vi "merFISH_save_embryo_position.vi"(6 "XY REF cluster":T1, 7 "queue ASI stage":refnum<queue>, 8 "error in":errorcluster, 9 "Image Dst":T2, 10 "Image contrast":cluster{i32, i32}, 11 "New Image":T2) -> (0 "error out":errorcluster, 3 "REF positions OUT":dbl[][](array[numeric]), 5 "XY positions OUT":dbl[][](array[numeric]))   [LabVIEW 2015]
uses:
  <vilib>/vision/Image Controls.llb/IMAQ Image.ctl
  CONTROLS/Q_ASI_stage_element.ctl
  GLOBAL/Global_ASI_stage.vi
panel:
  in  "Define REF":bool caption="Save X/Y position"
  in  "Define embryo":bool caption="Save X/Y position"
  in  "Embryo Pos 2":bool caption="Save X/Y position"
  in  "Embryo Pos 1":bool caption="Save X/Y position"
  out "XY positions":cluster{dbl[], dbl[]}[](graph)
  in  "stop":bool
  out "Intensity range":cluster{sgl, sgl}(slide) scale=0.0..16000.0
  out "Image":T2(plugin-control)
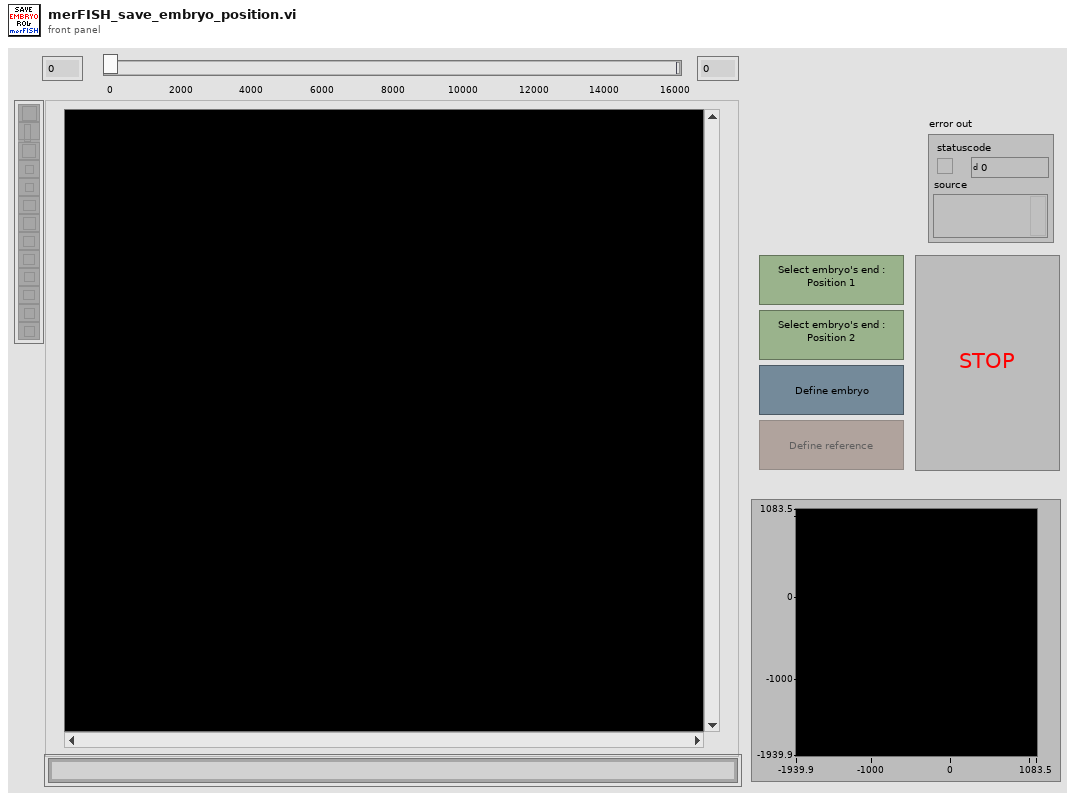
[diagram p1: front panel]
types:
  T1 = cluster{"XY positions":dbl[][], "REF positions":dbl[][]}
  T2 = typedef "IMAQ Image.ctl" = refnum<image>
  T3 = enum8{"Enabled", "Disabled", "Disabled and Grayed Out"}
  T4 = cluster{"Left":i32, "Top":i32, "Right":i32, "Bottom":i32}
  T5 = typedef "Q_ASI_stage_element.ctl" = cluster{"variant":variant, "Instruction":enum16{"ASI_idle", "ASI_initialize", "ASI_error", "ASI_security_stop", "ASI_read_XYZ", "ASI_up", "ASI_down", "ASI_left", "ASI_right", "ASI_save_XY", "ASI_move_to_XY", "ASI_brightfield", "ASI_init_scan", "ASI_init_merFISH", "ASI_move_to_XY_merFISH", "ASI_move_to_Z_merFISH", "ASI_init_autofocus_search_merFISH", "ASI_close_autofocus_search_merFISH", "ASI_adjust_piezo_autofocus_merFISH", "ASI_set_piezo_autofocus_to_reference_position_merFISH_TL", "ASI_close_merFISH", "ASI_stop"}}
  T6 = cluster{"Mean Value":sgl, "Standard Variation":sgl, "Minimal Value":sgl, "Maximal Value":sgl, "Area (calibrated)":sgl, "Area (pixels)":u32, "%":sgl, "Calibration Valid":bool}
  T7 = cluster{"Maximal Value":sgl, "Minimal Value":sgl}
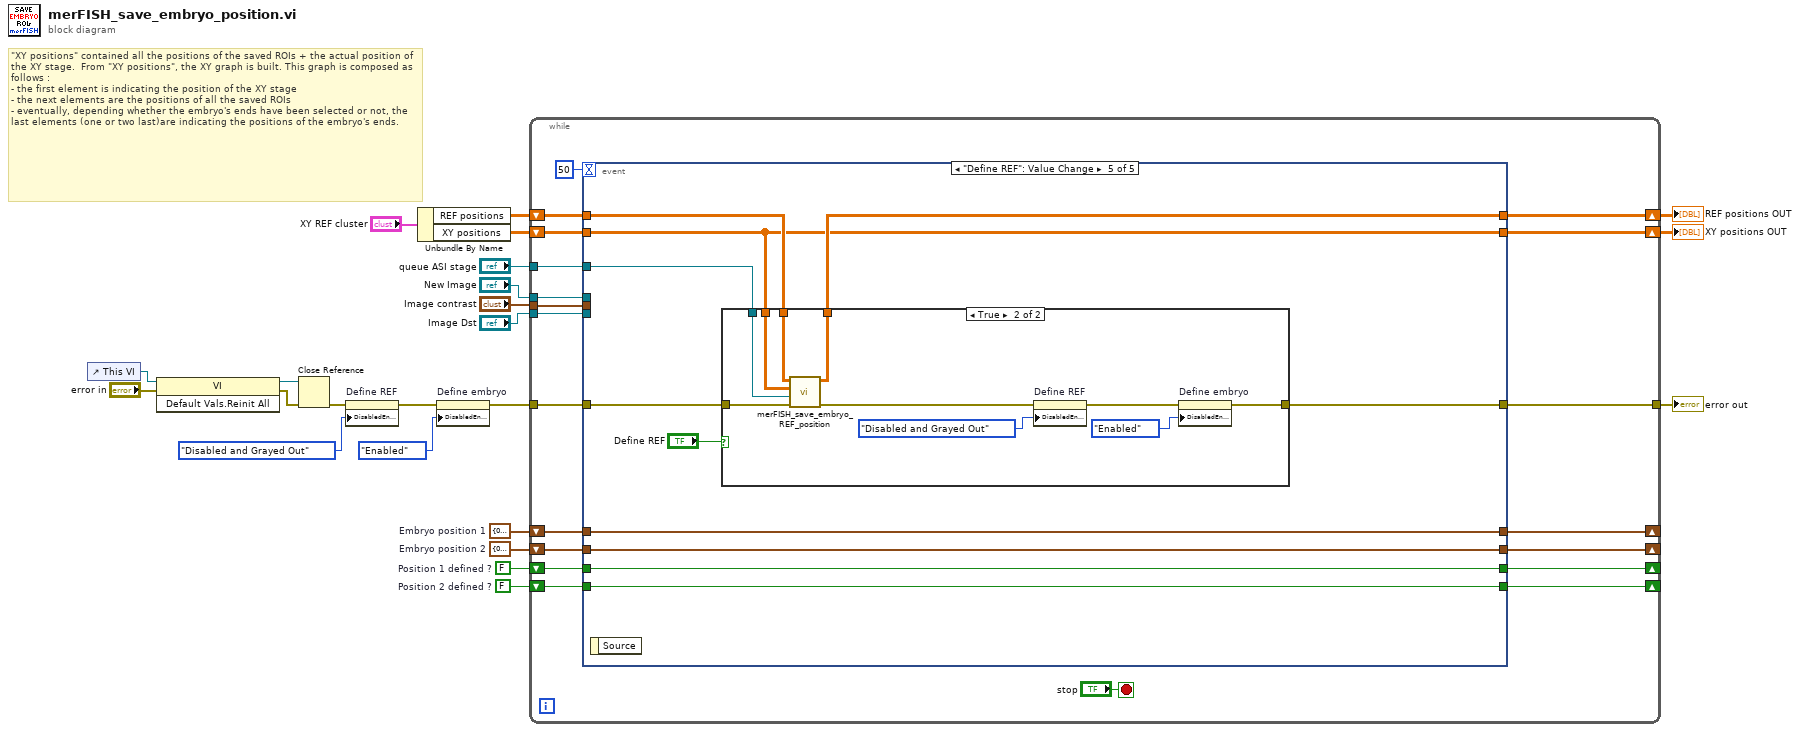
[diagram p0: block diagram]
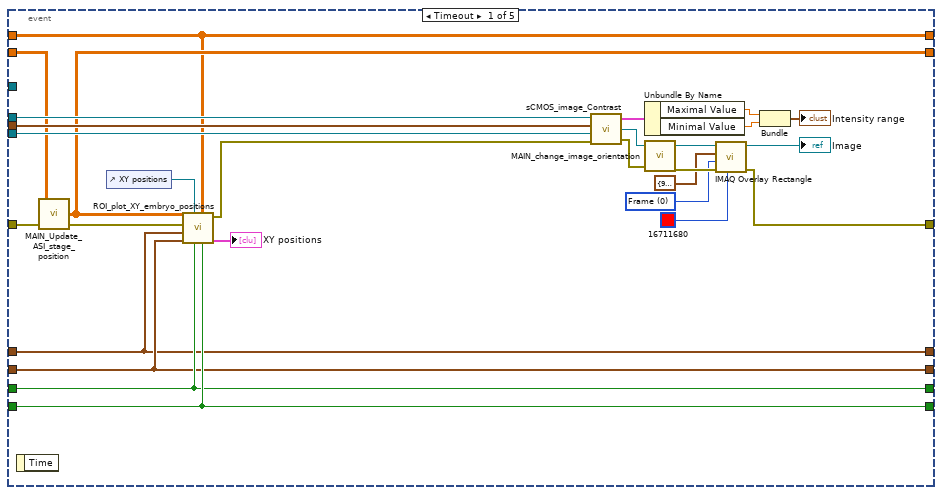
[diagram p2: hidden frame]
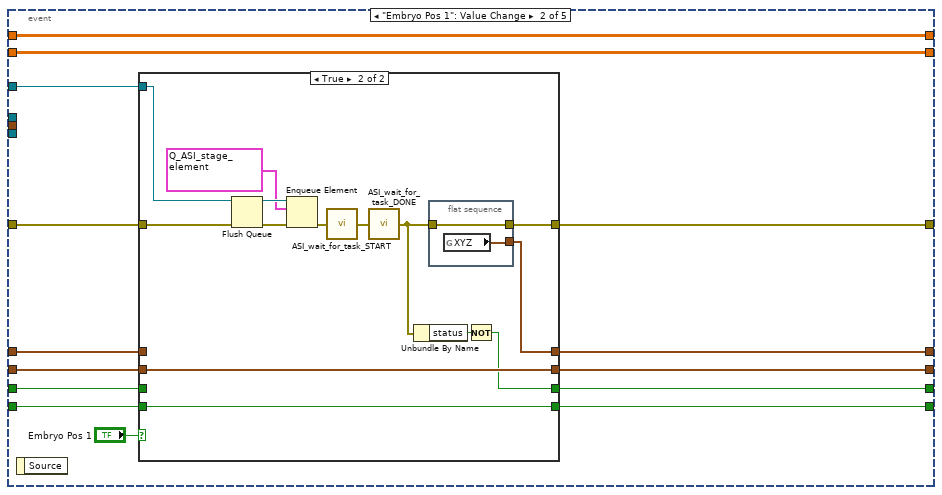
[diagram p3: hidden frame]
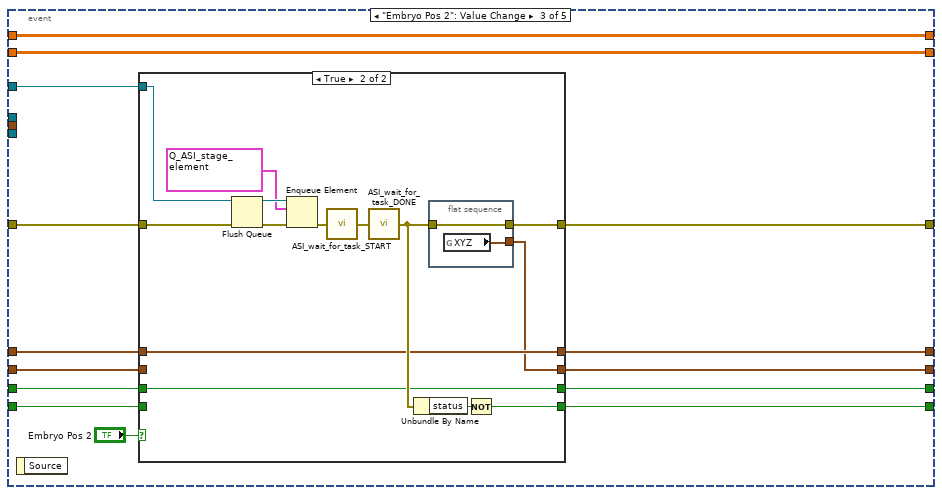
[diagram p5: hidden frame]
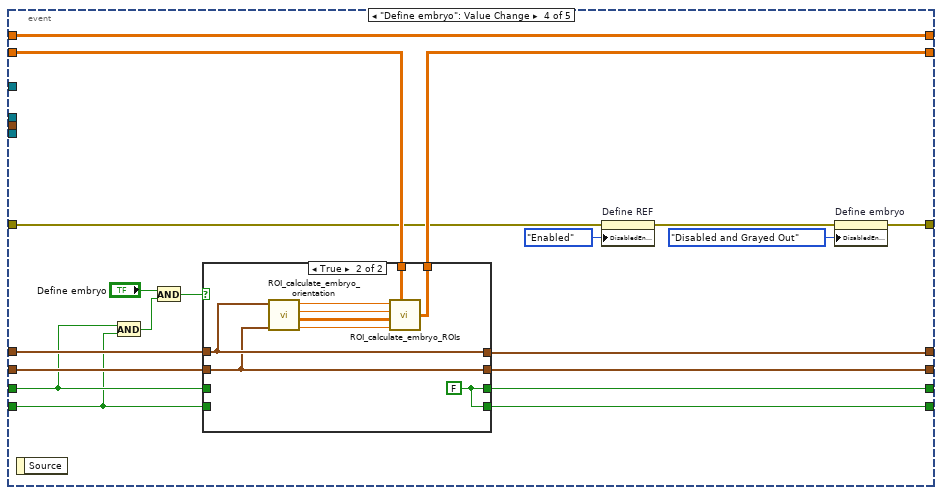
[diagram p7: hidden frame]
diagram:
  w12 = FALSE  # Position 2 defined ?
  w13 = FALSE  # Position 1 defined ?
  w14 = cluster{"x(um)":dbl, "y(um)":dbl, "z(um)":dbl} {"x(um)"=0.0, "y(um)"=0.0, "z(um)"=0.0}  # Embryo position 2
  w15 = cluster{"x(um)":dbl, "y(um)":dbl, "z(um)":dbl} {"x(um)"=0.0, "y(um)"=0.0, "z(um)"=0.0}  # Embryo position 1
  # "\"XY positions\" contained all the positions of the saved ROIs + the actual position of the XY stage.  From \"XY positions\", the XY graph is built. This graph is composed as follows :\n- the first element is indicating the position of the XY stage\n- the next elements are the positions of all the saved ROIs\n- eventually, depending whether the embryo's ends have been selected or not, the last elements (one or two last)are indicating the positions of the embryo's ends."
  n1 = control-ref of="This VI"() -> (w20:refnum<vi>)
  n2 = invoke class="VI" method="Default Vals.Reinit All"(reference=w20, error in="error in") -> (reference out=w19:refnum<vi>, error out=w18:errorcluster)  [unwired: 1 in, 1 out]
  n3 = Close Reference(reference=w19, error in (no error)=w18) -> (error out=w9:errorcluster)
  n4 = property on="Define REF" class="Bool (strict)"(error in=w9, "DisabledEnum"=T3."Disabled and Grayed Out" ("Disabled")) -> (error out=w7:errorcluster)  [unwired: 1 in, 1 out]
  n5 = Unbundle By Name("XY REF cluster") -> ("REF positions"=w2:dbl[][], "XY positions"=w1:dbl[][])
  n6 = property on="Define embryo" class="Bool (strict)"(error in=w7, "DisabledEnum"=T3."Enabled" ("Disabled")) -> (error out=w5:errorcluster)  [unwired: 1 in, 1 out]
  n7 = while {
    tunnel: "Image contrast" -> [w43]
    tunnel: "New Image" -> [w42]
    tunnel: "Image Dst" -> [w41]
    tunnel: "queue ASI stage" -> [w36]
    shift-right: [w32] -> _
    shift-left: w15 -> [w35]
    shift-right: [w33] -> _
    shift-left: w14 -> [w34]
    shift-right: [w29] -> _
    shift-left: w13 -> [w31]
    shift-right: [w28] -> _
    shift-left: w12 -> [w30]
    shift-right: [w26] -> w10
    shift-left: w1 -> [w27]
    shift-right: [w24] -> w4
    shift-left: w2 -> [w25]
    tunnel: w5 -> [w38]
    tunnel: [w39] -> w17
    stop <- "stop" stop-if-true
    n8 = event shown="[4] \"Define REF\": Value Change" {
      selector: _ -> [_ _ _ _ _]
      dyn-events: _ -> [_ _ _ _ _]
      timeout: 50 -> [_ _ _ _ _]
      tunnel: w43 -> [w65 _ _ _ _]
      tunnel: w42 -> [w64 _ _ _ _]
      tunnel: w41 -> [w63 _ _ _ _]
      tunnel: [w56 w82 w117 w143 w185] -> w39
      tunnel: w38 -> [w55 w84 w119 w147 w180]
      tunnel: w36 -> [_ w83 w118 _ w179]
      tunnel: w35 -> [w48 w78 w113 w160 w184]
      tunnel: w34 -> [w49 w80 w115 w159 w183]
      tunnel: [w49 w81 w116 w148 w183] -> w33
      tunnel: [w48 w79 w114 w149 w184] -> w32
      tunnel: w31 -> [w50 w76 w109 w153 w182]
      tunnel: w30 -> [w51 w75 w111 w152 w181]
      tunnel: [w50 w77 w110 w150 w182] -> w29
      tunnel: [w51 w74 w112 w151 w181] -> w28
      tunnel: w27 -> [w52 w73 w108 w158 w175]
      tunnel: [w46 w73 w108 w157 w175] -> w26
      tunnel: w25 -> [w44 w72 w107 w142 w178]
      tunnel: [w44 w72 w107 w142 w177] -> w24
      event Timeout {
        w59 = u32 0 items=["Frame", "Fill", "Highlight"] ("Drawing Mode (Frame)")
        n9 = event-data() -> ()  [unwired: 1 in, 1 out]
        n10 = call "MAIN_Update_ASI_stage_position.vi"("error in"=w55, "XY positions"=w52) -> ("error out"=w47:errorcluster, "XY positions OUT"=w46:dbl[][])  [unwired: 1 in, 1 out]
        n11 = control-ref of="XY positions"() -> (w45:refnum<vi>)
        n12 = call "ROI_plot_XY_embryo_positions.vi"("Pos 2 saved"=w51, "REF positions"=w44, "Pos 1 saved"=w50, "XYGraph Refnum"=w45, "Embryo position 2"=w49, "Embryo position 1"=w48, "error in"=w47, "XY positions"=w46) -> ("XY graph"=→"XY positions":cluster{dbl[], dbl[]}[], "error out"=w53:errorcluster)  [unwired: 2 in]
        n13 = call "sCMOS_image_Contrast.vi"("error in"=w53, "Image Dst"=w63, "Image contrast"=w65, "New Image"=w64) -> ("error out"=w68:errorcluster, "Image Dst Out"=w67:T2, "Global Report"=w71:T6)
        n14 = Unbundle By Name(w71) -> ("Maximal Value"=w70:sgl, "Minimal Value"=w69:sgl)
        n15 = call "MAIN_change_image_orientation.vi"("error in"=w68, "Image IN"=w67) -> ("error out"=w61:errorcluster, "Image Out"=w62:T2)  [unwired: 2 in]
        n16 = call "IMAQ Overlay Rectangle"("Color"=u32 16711680, "error in (no error)"=w61, "Drawing Mode (Frame)"=w59, "Rectangle"=T4 {"Left"=974, "Top"=974, "Right"=1074, "Bottom"=1074}, "Image"=w62) -> ("error out"=w56:errorcluster, "Image Out"=→"Image":T2)  [unwired: 5 in]
        n17 = Bundle("Maximal Value"=w70, "Minimal Value"=w69) -> (→"Intensity range":T7)  [unwired: 1 in]
      }
      event "Embryo Pos 1": Value Change {
        n18 = event-data() -> ()  [unwired: 1 in, 1 out]
        n19 = case shown="True" "Embryo Pos 1" {
          tunnel: w84 -> [w90 w99]
          tunnel: w83 -> [_ w98]
          tunnel: [w90 w93] -> w82
          tunnel: [w88 w95] -> w81
          tunnel: w80 -> [w88 w95]
          tunnel: [w89 w94] -> w79
          tunnel: w78 -> [w89 _]
          tunnel: [w87 w92] -> w77
          tunnel: w76 -> [w87 _]
          tunnel: w75 -> [w86 w91]
          tunnel: [w86 w91] -> w74
          frame False {
          }
          frame True {
            n20 = Flush Queue(queue=w98, error in (no error)=w99) -> (queue out=w104:refnum<queue>, error out=w103:errorcluster)  [unwired: 1 out]
            n21 = Enqueue Element(queue=w104, element=T5 {"variant"=variant, "Instruction"=enum."ASI_save_XY"} ("Q_ASI_stage"), error in (no error)=w103) -> (error out=w101:errorcluster)  [unwired: 1 in, 2 out]
            n22 = call "ASI_wait_for_task_START.vi"("error in"=w101) -> ("error out"=w100:errorcluster)
            n23 = call "ASI_wait_for_task_DONE.vi"("error in"=w100) -> ("error out"=w96:errorcluster)
            n24 = Unbundle By Name(w96) -> ("status"=w97:bool)
            n25 = flat-sequence {
              tunnel: w96 -> [w105]
              tunnel: [w106] -> w94
              tunnel: [w105] -> w93
              frame #0 {
                n26 = global read "Global_ASI_stage.vi" "XYZ"() -> (w106:cluster{"x(um)":dbl, "y(um)":dbl, "z(um)":dbl})
              }
            }
            n27 = Not(x=w97) -> (.not. x?=w92:bool)
          }
        }
      }
      event "Embryo Pos 2": Value Change {
        n28 = event-data() -> ()  [unwired: 1 in, 1 out]
        n29 = case shown="True" "Embryo Pos 2" {
          tunnel: w119 -> [w125 w134]
          tunnel: w118 -> [_ w133]
          tunnel: [w125 w130] -> w117
          tunnel: [w123 w128] -> w116
          tunnel: w115 -> [w123 _]
          tunnel: [w124 w129] -> w114
          tunnel: w113 -> [w124 w129]
          tunnel: [w122 w127] -> w112
          tunnel: w111 -> [w122 _]
          tunnel: [w121 w126] -> w110
          tunnel: w109 -> [w121 w126]
          frame False {
          }
          frame True {
            n30 = Flush Queue(queue=w133, error in (no error)=w134) -> (queue out=w139:refnum<queue>, error out=w138:errorcluster)  [unwired: 1 out]
            n31 = Enqueue Element(queue=w139, element=T5 {"variant"=variant, "Instruction"=enum."ASI_save_XY"} ("Q_ASI_stage"), error in (no error)=w138) -> (error out=w136:errorcluster)  [unwired: 1 in, 2 out]
            n32 = call "ASI_wait_for_task_START.vi"("error in"=w136) -> ("error out"=w135:errorcluster)
            n33 = call "ASI_wait_for_task_DONE.vi"("error in"=w135) -> ("error out"=w131:errorcluster)
            n34 = Unbundle By Name(w131) -> ("status"=w132:bool)
            n35 = flat-sequence {
              tunnel: w131 -> [w140]
              tunnel: [w141] -> w128
              tunnel: [w140] -> w130
              frame #0 {
                n36 = global read "Global_ASI_stage.vi" "XYZ"() -> (w141:cluster{"x(um)":dbl, "y(um)":dbl, "z(um)":dbl})
              }
            }
            n37 = Not(x=w132) -> (.not. x?=w127:bool)
          }
        }
      }
      event "Define embryo": Value Change {
        n38 = event-data() -> ()  [unwired: 1 in, 1 out]
        n39 = And(x=w153, y=w152) -> (x .and. y?=w154:bool)
        n40 = And(x="Define embryo", y=w154) -> (x .and. y?=w155:bool)
        n41 = case shown="True" w155 {
          tunnel: w160 -> [w162 w167]
          tunnel: w159 -> [w161 w166]
          tunnel: w158 -> [w165 w170]
          tunnel: [w165 w169] -> w157
          tunnel: w153 -> [w164 _]
          tunnel: w152 -> [w163 _]
          tunnel: [w163 w168] -> w151
          tunnel: [w164 w168] -> w150
          tunnel: [w162 w167] -> w149
          tunnel: [w161 w166] -> w148
          frame False {
          }
          frame True {
            w168 = FALSE ("Position 1 defined ?")
            n42 = call "ROI_calculate_embryo_orientation.vi"("Embryo position 2"=w166, "Embryo position 1"=w167) -> ("Slope a"=w171:dbl, "Embryo's ends"=w172:dbl[][], "b"=w173:dbl, "Angle"=w174:dbl)  [unwired: 2 in]
            n43 = call "ROI_calculate_embryo_ROIs.vi"("Angle"=w174, "b"=w173, "Embryo's ends"=w172, "Slope a"=w171, "XY positions"=w170) -> ("ROIs"=w169:dbl[][])
          }
        }
        n44 = property on="Define REF" class="Bool (strict)"(error in=w147, "DisabledEnum"=T3."Enabled" ("Disabled")) -> (error out=w145:errorcluster)  [unwired: 1 in, 1 out]
        n45 = property on="Define embryo" class="Bool (strict)"(error in=w145, "DisabledEnum"=T3."Disabled and Grayed Out" ("Disabled")) -> (error out=w143:errorcluster)  [unwired: 1 in, 1 out]
      }
      event "Define REF": Value Change {
        n46 = event-data() -> ()  [unwired: 1 in, 1 out]
        n47 = case shown="True" "Define REF" {
          tunnel: [w186 w195] -> w185
          tunnel: w180 -> [w186 w193]
          tunnel: w179 -> [_ w191]
          tunnel: w178 -> [w187 w190]
          tunnel: [w187 w189] -> w177
          tunnel: w175 -> [_ w188]
          frame False {
          }
          frame True {
            n48 = call "merFISH_save_embryo_REF_position.vi"("error in"=w193, "queue ASI stage"=w191, "ROI positions"=w188, "REF positions"=w190) -> ("error out"=w192:errorcluster, "REF positions OUT"=w189:dbl[][])  [unwired: 2 in]
            n49 = property on="Define REF" class="Bool (strict)"(error in=w192, "DisabledEnum"=T3."Disabled and Grayed Out" ("Disabled")) -> (error out=w196:errorcluster)  [unwired: 1 in, 1 out]
            n50 = property on="Define embryo" class="Bool (strict)"(error in=w196, "DisabledEnum"=T3."Enabled" ("Disabled")) -> (error out=w195:errorcluster)  [unwired: 1 in, 1 out]
          }
        }
      }
    }
  }
  "error out" <- w17
  "XY positions OUT" <- w10
  "REF positions OUT" <- w4
